vi "PH_AxisGUI_6P.PC_Settings.vi"(0 "i ref in":refnum<vi>, 1 "Service Name":string, 2 "Axis Settings":T2={"Sign change"=FALSE, "Width"=0.0, "Calibration Factor"=0.0, "Unit"="Steps", "Motor Type"=enum."Unspecific"}, 5 "error in":errorcluster) -> (14 "i ref out":refnum<vi>, 15 "Axis Selector":T1, 16 "Unit":string, 19 "error":errorcluster)   [LabVIEW 2014]
uses:
  PH_AxisGUI_6P.lvlib
  PH_AxisGUI_BaseClass/PH_AxisGUI_BaseClass.lvlib
  PH_AxisGUI_6P.AxisSelector.ctl
  PH_Common/PH_Motion/PH_Motion.Motor Type.ctl
  PH_Common/PH_Motion/PH_Motion.Axis Settings.ctl
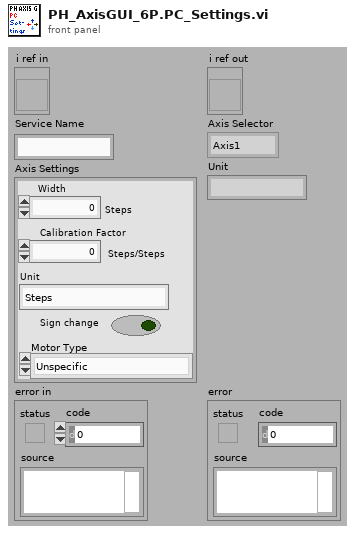
[diagram p1: front panel]
types:
  T1 = typedef "PH_AxisGUI_6P.lvlib/PH_AxisGUI_6P.AxisSelector.ctl" = enum16{"Axis1", "Axis2", "None"}
  T2 = typedef "PH_Motion.Axis Settings.ctl" = cluster{"Sign change":bool, "Width":dbl, "Calibration Factor":dbl, "Unit":string, "Motor Type":T3}
  T3 = typedef "PH_Motion.Motor Type.ctl" = enum16{"Unspecific", "OWIS 49.120.2633", "OWIS 49.060.1033", "OWIS 43.040.2558", "Diamond Motion 2200 series", "OWIS 49.120.266B.MV6", "Calorimeter", "Linear Stage 1", "MICOS VT-80", "MICOS VT-80 S", "Standa Rotstage nt0.95A", "PUF RA 320.200", "PUF RA 800.200", "PUF RA 800.400", "PUF RA 400.50", "1324.nn.800.50", "1324.n9c.800.50"}
  T4 = typedef "PH_AxisGUI_6P.lvlib/PH_AxisGUI_6P.i attribute.ctl" = cluster{"GUI Refs":cluster{"AxisSelection":refnum<vi>, "Tab Control":refnum<vi>}}
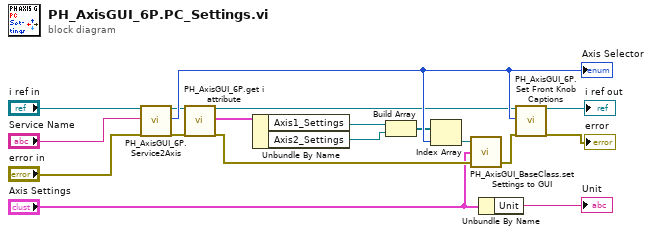
[diagram p0: block diagram]
diagram:
  n1 = call "PH_AxisGUI_6P.Service2Axis.vi"("i ref in"="i ref in", "service name"="Service Name", "error in"="error in") -> ("i ref out"=w12:refnum<vi>, "Axis Selector"=w14:T1, "error out"=w11:errorcluster)  [unwired: 14 in]
  "Axis Selector" <- w14
  n2 = call "PH_AxisGUI_6P.get i attribute.vi"("i ref in"=w12, "error in (no error)"=w11) -> ("i ref out"=w3:refnum<vi>, "i attribute"=w5:T4, "error out"=w7:errorcluster)  [unwired: 15 in]
  n3 = Unbundle By Name(w5) -> ("Axis1_Settings"=w10:refnum<vi>, "Axis2_Settings"=w9:refnum<vi>)
  n4 = Build Array(w10, w9) -> (w8:refnum<vi>[])
  n5 = Index Array(array=w8, index=w14) -> (element=w6:refnum<vi>)
  n6 = call "PH_AxisGUI_BaseClass.set Settings to GUI.vi"("error in (no error)"=w7, "Axis Settings"="Axis Settings", "GUI Ref Settings"=w6) -> ("error out"=w4:errorcluster)  [unwired: 2 in]
  n7 = Unbundle By Name("Axis Settings") -> ("Unit"=→"Unit":string)
  n8 = call "PH_AxisGUI_6P.Set Front Knob Captions.vi"("i ref out"=w3, "Axis Selector"=w14, "error in"=w4) -> ("i ref out"=→"i ref out":refnum<vi>, "error out"=→"error":errorcluster)  [unwired: 15 in]
